vi "ProWave.vi"() -> ()   [LabVIEW 2019]
uses:
  <vilib>/rvi/Emulation/niFpgaGetClockAttributes.vi
  <vilib>/rvi/Emulation/niFpgaSctlEmulationGetInTimedLoop.vi
  <vilib>/rvi/Emulation/niFpgaEmulationReportErrorSimple.vi
  <vilib>/rvi/eio/common/nirviEmuTemplateMethod_errors.vi
  <vilib>/rvi/Emulation/niFpgaCriticalErrorInLSC.vi
  <vilib>/eio/EIONode/EIONode.xnode
panel:
  in  "当前转速":fxp<+,64,32>
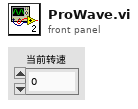
[diagram p1: front panel]
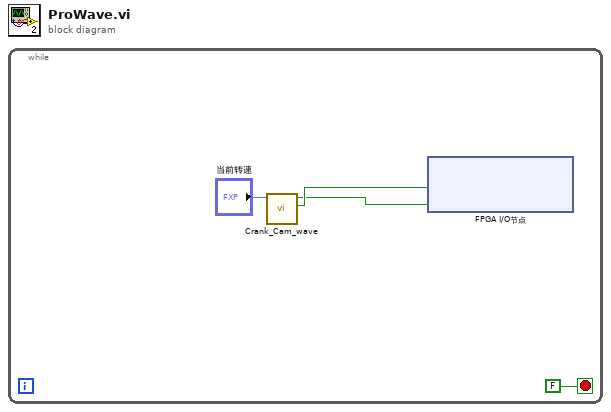
[diagram p0: block diagram]
diagram:
  n1 = while {
    stop <- FALSE stop-if-true
    n2 = call "Crank_Cam_wave.vi"("当前转速"="当前转速") -> ("曲轴"=w3:bool, "凸轮轴"=w2:bool)  [unwired: 9 in]
    n3 = xnode "FPGA I/O节点"("Connector0/DIO0"=w3, "Connector0/DIO1"=w2) -> ()  [unwired: 2 in, 2 out]
  }
